vi "Get Time.vi"(8 "error in (no error)":errorcluster, 11 "Event in":refnum<class "Event.lvclass">) -> (0 "error out":errorcluster, 2 "Time out":refnum<class "Uint64.lvclass">, 3 "Event out":refnum<class "Event.lvclass">)   [LabVIEW 2010, in "MDSplus.lvlib" / "Event.lvclass"]
doc: "Return data received last."
uses:
  <vilib>/MDSplus/Classes/Event_Class/Event.lvclass
  <vilib>/MDSplus/Classes/Data_Class/Scalar_Class/Uint64_Class/Uint64.lvclass
  <vilib>/MDSplus/Classes/Data_Class/Data.lvclass
  <vilib>/MDSplus/MDSobjectsLVShr.dll
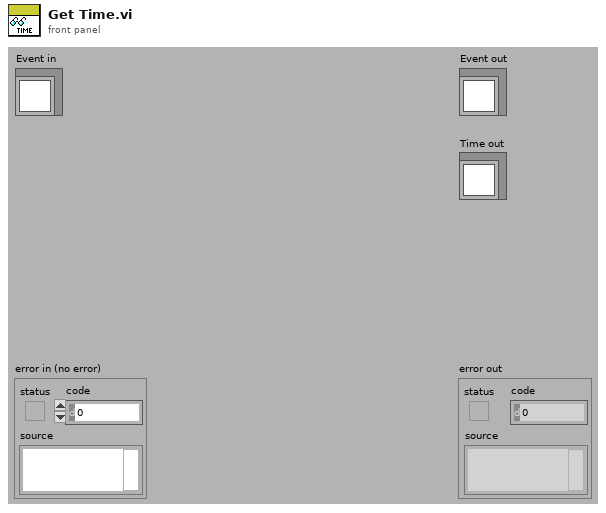
[diagram p1: front panel]
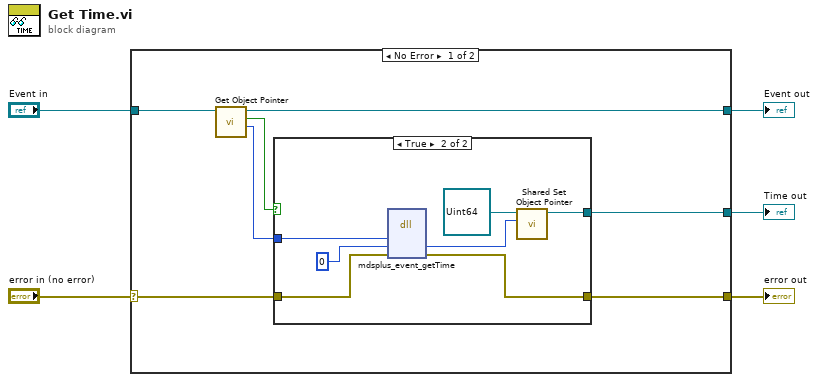
[diagram p0: block diagram]
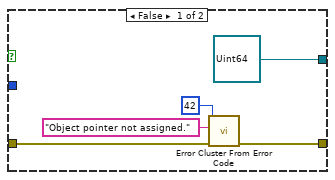
[diagram p2: hidden frame]
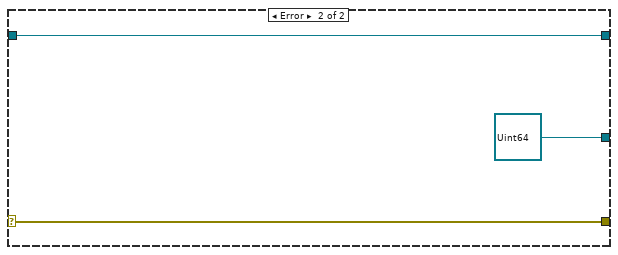
[diagram p3: hidden frame]
diagram:
  n1 = case shown="No Error" "error in (no error)" {
    selector: "error in (no error)" -> [w8 w27]
    tunnel: [w7 w27] -> w4
    tunnel: [w6 w26] -> w2
    tunnel: "Event in" -> [w11 w26]
    tunnel: [w12 refnum<class "Uint64.lvclass"> refnum ("Data out")] -> w1
    frame No Error {
      n2 = call-dynamic "Get Object Pointer.vi"("Event in"=w11) -> ("Object Pointer"=w9:i64, "Assigned object pointer?"=w10:bool, "Event out"=w6:refnum<class "Event.lvclass">)  [unwired: 8 in]
      n3 = case shown="True" w10 {
        tunnel: [refnum<class "Uint64.lvclass"> refnum ("Data out") w19] -> w12
        tunnel: w9 -> [_ w21]
        tunnel: w8 -> [w14 w20]
        tunnel: [w13 w18] -> w7
        frame False {
          n4 = call <vilib>:"Error Cluster From Error Code.vi"("error in (no error)"=w14, "error message (\"\")"="Object pointer not assigned." ("error message (\"\")"), "error code (0)"=42) -> ("error out"=w13:errorcluster)  [unwired: 6 in]
        }
        frame True {
          n5 = dll-call lib="C:/Program Files/National Instruments/LabVIEW 2010/vi.lib/MDSplus/MDSobjectsLVShr**.*" fn="mdsplus_event_getTime"("lvEventPtr"=w21, "lvUint64PtrOut"=i64 0 ("lvDataPtrOut"), "error"=w20) -> ("lvUint64PtrOut"=w22:i64, "error"=w18:errorcluster)  [unwired: 5 in, 2 out]
          n6 = call <vilib>:"Shared Set Object Pointer.vi"("Object Pointer"=w22, "Data in"=refnum<class "Uint64.lvclass"> refnum ("Uint64.lvclass")) -> ("Data out"=w19:refnum<class "Uint64.lvclass">)  [unwired: 9 in]
        }
      }
    }
    frame Error {
    }
  }
  "error out" <- w4
  "Event out" <- w2
  "Time out" <- w1
